vi "Initial Values-Compare-Boolean.vi"(5 "Function (Add)":T3=enum."Add", 7 "Current values":bool[](array[boolean]), 8 "error in (no error)":errorcluster, 9 "Keys Array":T2, 10 "Section name":string, 11 "User profile ini file ref":T5) -> (0 "error out":errorcluster, 1 "Keys of changed parameters":T1, 2 "Changed parameters info":T4[](array[typedef]), 3 "User profile ini file ref":T5, 4 "Changes exist":bool)   [LabVIEW 2013]
uses:
  <vilib>/Utility/config.llb/Config Data RefNum.ctl
  User Interface/User profiles code/Typedefs/Changed parameter cluster.ctl
  User Interface/User profiles code/Typedefs/Comparison states.ctl
  Typedefs/Ini file interface (Boolean).ctl
  User Interface/User profiles code/Typedefs/Changes info cluster-BOOL.ctl
  Program Files (x86)/National Instruments/LabVIEW 2013/user.lib/_OpenG.lib/array/array.llb/Search 1D Array (Boolean)__ogtk.vi
  Program Files (x86)/National Instruments/LabVIEW 2013/user.lib/_OpenG.lib/array/array.llb/Index 1D Array Elements (Boolean)__ogtk.vi
  Program Files (x86)/National Instruments/LabVIEW 2013/user.lib/_OpenG.lib/array/array.llb/Index 1D Array Elements (Variant)__ogtk.vi
  <vilib>/Utility/config.llb/NI_LVConfig.lvlib
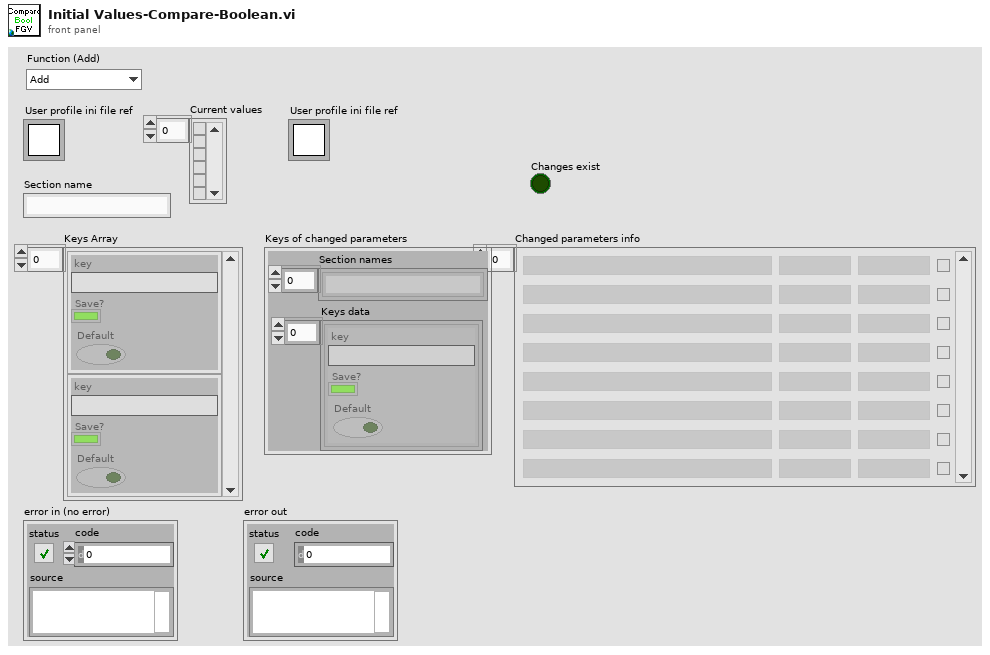
[diagram p1: front panel]
types:
  T1 = typedef "Changes info cluster-BOOL.ctl" = cluster{"Section names":string[], "Keys data":T2}
  T2 = typedef "Ini file interface (Boolean).ctl" = cluster{"key":string, "Save?":bool, "Default":bool}[]
  T3 = typedef "Comparison states.ctl" = enum16{"Init.", "Add", "Read"}
  T4 = typedef "Changed parameter cluster.ctl" = cluster{"Name":string, "Old value":string, "New value":string, "Save":bool}
  T5 = typedef "NI_LVConfig.lvlib/Config Data RefNum.ctl" = refnum<k1>
  T6 = cluster{"key":string, "Save?":bool, "Default":bool}[]
  T7 = cluster{"key":string, "Save?":bool, "Default":bool}
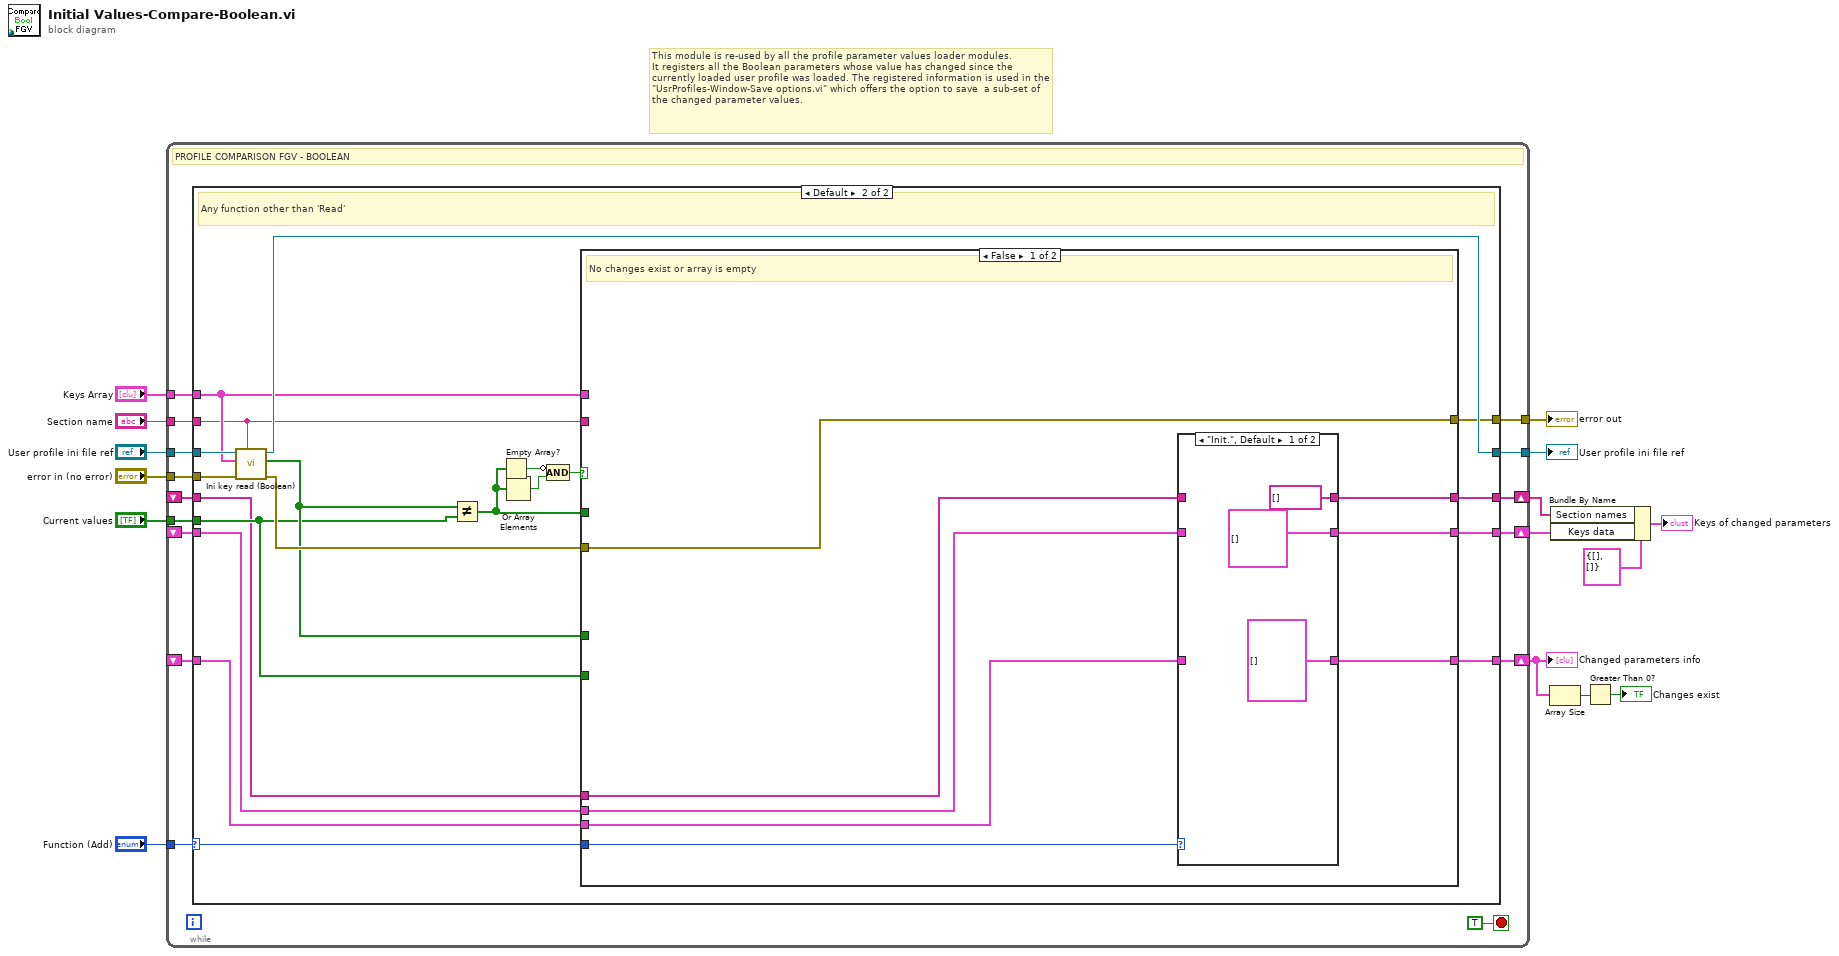
[diagram p0: block diagram]
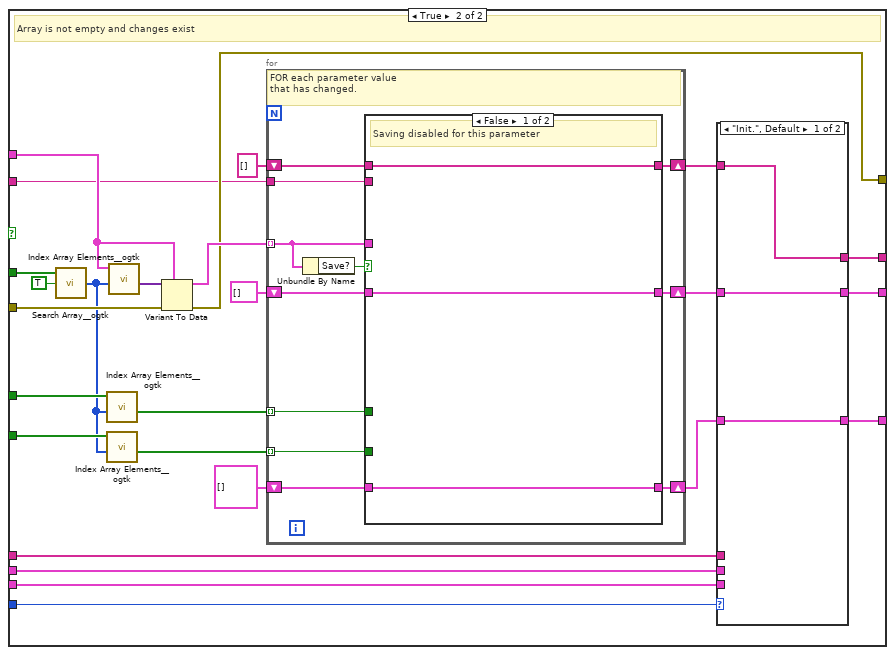
[diagram p4: hidden frame]
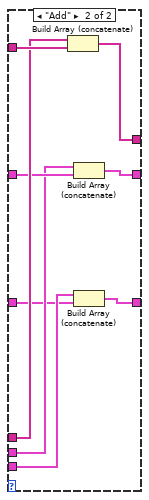
[diagram p5: hidden frame]
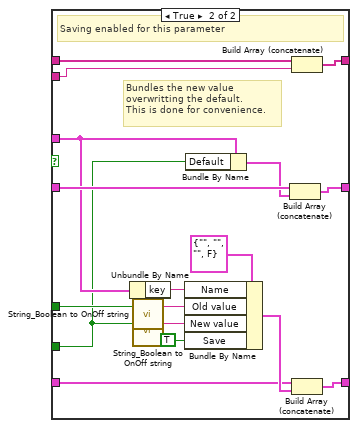
[diagram p6: hidden frame]
diagram:
  # "This module is re-used by all the profile parameter values loader modules.\nIt registers all the Boolean parameters whose value has changed since the currently loaded user profile was loaded. The registered information is used in the \"UsrProfiles-Window-Save options.vi\" which offers the option to save  a sub-set of the changed parameter values."
  n1 = while {
    tunnel: "Section name" -> [w30]
    tunnel: "error in (no error)" -> [w29]
    tunnel: [w28] -> w13
    tunnel: "User profile ini file ref" -> [w27]
    tunnel: "Keys Array" -> [w26]
    tunnel: "Current values" -> [w19]
    tunnel: [w24] -> w10
    shift-right: [w20] -> w2
    shift-left: _ -> [w22]
    shift-right: [w23] -> w6
    shift-left: _ -> [w21]
    tunnel: "Function (Add)" -> [w18]
    shift-right: [w17] -> w1
    shift-left: _ -> [w16]
    stop <- TRUE stop-if-true
    # "PROFILE COMPARISON FGV - BOOLEAN"
    n2 = case shown="Default" w18 {
      selector: w18 -> [_ w39]
      tunnel: w30 -> [_ w38]
      tunnel: w29 -> [w34 w55]
      tunnel: [w35 w54] -> w28
      tunnel: w27 -> [w35 w53]
      tunnel: w26 -> [_ w52]
      tunnel: [w34 w50] -> w24
      tunnel: [w32 w49] -> w23
      tunnel: w22 -> [w33 w48]
      tunnel: w21 -> [w32 w47]
      tunnel: [w33 w43] -> w20
      tunnel: w19 -> [_ w41]
      tunnel: [w31 w37] -> w17
      tunnel: w16 -> [w31 w36]
      frame "Read" {
        # "The selected function is 'Read'"
      }
      frame Default {
        # "Any function other than 'Read'"
        n3 = call "Ini key read (Boolean).vi"("Section"=w38, "error in (no error)"=w55, "Parameter names & setup"=w52, "Ini file refnum in"=w53) -> ("error out"=w51:errorcluster, "Value read/used"=w42:bool[], "Ini file refnum out"=w54:T5)  [unwired: 5 in]
        n4 = Not Equal?(x=w42, y=w41) -> (x != y?=w40:bool[])
        n5 = Empty Array?(array=w40) -> (empty?=w46:bool)
        n6 = Or Array Elements(Boolean array=w40) -> (logical OR=w45:bool)
        n7 = Compound Arithmetic op=AND(invert w46, w45) -> (w44:bool)
        n8 = case shown="False" w44 {
          tunnel: w52 -> [_ w95]
          tunnel: w41 -> [_ w94]
          tunnel: w40 -> [_ w93]
          tunnel: w51 -> [w63 w90]
          tunnel: w42 -> [_ w89]
          tunnel: w39 -> [w59 w84]
          tunnel: [w63 w77] -> w50
          tunnel: [w60 w81] -> w49
          tunnel: w48 -> [w62 w80]
          tunnel: w47 -> [w61 w79]
          tunnel: [w56 w75] -> w43
          tunnel: w38 -> [_ w74]
          tunnel: [w57 w71] -> w37
          tunnel: w36 -> [w58 w70]
          frame False {
            # "No changes exist or array is empty"
            n9 = case shown="\"Init.\", Default" w59 {
              tunnel: w62 -> [_ w68]
              tunnel: w61 -> [_ w69]
              tunnel: [T4[] [] w69] -> w60
              tunnel: [T2 [] ("Keys of changed parameters") w68] -> w56
              tunnel: [string[] [] w67] -> w57
              tunnel: w58 -> [_ w67]
              frame "Init.", Default {
              }
              frame "Add" {
              }
            }
          }
          frame True {
            # "Array is not empty and changes exist"
            n10 = call-poly "Search Array__ogtk.vi"("Array"=w93, "Element Data"=TRUE) -> ("Indices of Elements"=w87:i32[])  [unwired: 7 in]
            n11 = call-poly "Index Array Elements__ogtk.vi"("indices"=w87, "array"=w89) -> ("elements"=w88:bool[])  [unwired: 9 in]
            n12 = call-poly "Index Array Elements__ogtk.vi"("indices"=w87, "array"=w94) -> ("elements"=w86:bool[])  [unwired: 9 in]
            n13 = call-poly "Index Array Elements__ogtk.vi"("indices"=w87, "array"=w95) -> ("elements"=w91:variant[])  [unwired: 9 in]
            n14 = Variant To Data(error in=w90, type=w95, Variant=w91) -> (data=w85:T2, error out=w77:errorcluster)
            n15 = for {
              tunnel: w88 -> [w118] mode=indexing
              tunnel: w86 -> [w117] mode=indexing
              tunnel: w85 -> [w114] mode=indexing
              shift-right: [w115] -> w83
              shift-left: T6 [] -> [w116]
              shift-right: [w113] -> w82
              shift-left: T4[] [] -> [w112]
              tunnel: w74 -> [w110]
              shift-right: [w109] -> w72
              shift-left: string[] [] -> [w108]
              # "FOR each parameter value\nthat has changed."
              n16 = Unbundle By Name(w114) -> ("Save?"=w111:bool)
              n17 = case shown="False" w111 {
                tunnel: w118 -> [_ w128]
                tunnel: w117 -> [_ w126]
                tunnel: w116 -> [w121 w135]
                tunnel: [w121 w133] -> w115
                tunnel: w114 -> [_ w132]
                tunnel: [w120 w130] -> w113
                tunnel: w112 -> [w120 w129]
                tunnel: w110 -> [_ w124]
                tunnel: [w119 w123] -> w109
                tunnel: w108 -> [w119 w122]
                frame False {
                  # "Saving disabled for this parameter"
                }
                frame True {
                  # "Bundles the new value\noverwritting the default.\nThis is done for convenience."
                  # "Saving enabled for this parameter"
                  n18 = Unbundle By Name(w132) -> ("key"=w136:string)
                  n19 = call "String_Boolean to OnOff string.vi"("Boolean value"=w128) -> ("ON/OFF string"=w127:string)  [unwired: 2 in]
                  n20 = call "String_Boolean to OnOff string.vi"("Boolean value"=w126) -> ("ON/OFF string"=w125:string)  [unwired: 2 in]
                  n21 = Bundle By Name(cluster=T4 {"Name"="", "Old value"="", "New value"="", "Save"=FALSE} ("Cluster"), "Name"=w136, "Old value"=w127, "New value"=w125, "Save"=TRUE) -> (w131:T4)
                  n22 = Bundle By Name(cluster=w132, "Default"=w126) -> (w134:T7)
                  n23 = Build Array (concatenate)(w135, w134) -> (w133:T6)
                  n24 = Build Array (concatenate)(w122, w124) -> (w123:string[])
                  n25 = Build Array (concatenate)(w129, w131) -> (w130:T4[])
                }
              }
            }
            n26 = case shown="\"Init.\", Default" w84 {
              tunnel: w83 -> [w97 w102]
              tunnel: w82 -> [w98 w99]
              tunnel: [w98 w107] -> w81
              tunnel: w80 -> [_ w101]
              tunnel: w79 -> [_ w100]
              tunnel: [w97 w106] -> w75
              tunnel: w72 -> [w96 w104]
              tunnel: [w96 w105] -> w71
              tunnel: w70 -> [_ w103]
              frame "Init.", Default {
              }
              frame "Add" {
                n27 = Build Array (concatenate)(w103, w104) -> (w105:string[])
                n28 = Build Array (concatenate)(w101, w102) -> (w106:T2)
                n29 = Build Array (concatenate)(w100, w99) -> (w107:T4[])
              }
            }
          }
        }
      }
    }
  }
  "User profile ini file ref" <- w13
  "error out" <- w10
  "Changed parameters info" <- w6
  n30 = Array Size(array=w6) -> (size(s)=w7:i32)
  n31 = Bundle By Name(cluster=T1 {"Section names"=[], "Keys data"=[]} ("Keys of changed parameters"), "Section names"=w1, "Keys data"=w2) -> (→"Keys of changed parameters":T1)
  n32 = Greater Than 0?(x=w7) -> (x > 0?=→"Changes exist":bool)
